vi "FinishMessage.vi"(4 "error":string="ERROR", 5 "no error":string="OK", 6 "error in":errorcluster, 9 "MessageBox in":refnum<class "MessageBox.lvclass">) -> (0 "error out":errorcluster, 3 "MessageBox out":refnum<class "MessageBox.lvclass">)   [LabVIEW 2014, in "MessageBox.lvclass"]
uses:
  MessageBox.lvclass
  MessageBox.lvclass/MessageBox.ctl
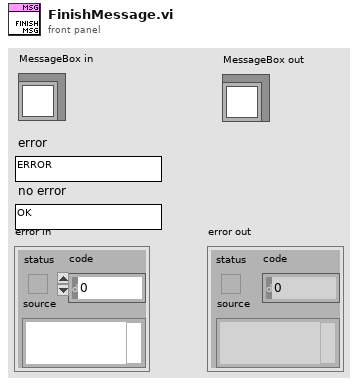
[diagram p1: front panel]
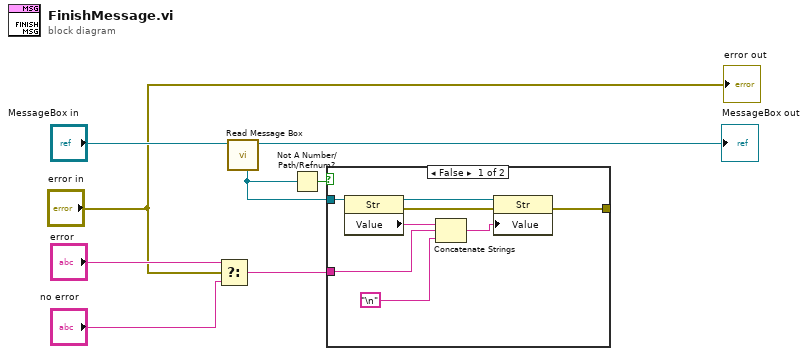
[diagram p0: block diagram]
diagram:
  n1 = Select(t="error", s="error in", f="no error") -> (s? t:f=w3:string)
  n2 = call "Read Message Box.vi"("MessageBox in"="MessageBox in") -> ("MessageBox out"=→"MessageBox out":refnum<class "MessageBox.lvclass">, "Message Box"=w5:refnum<vi>)  [unwired: 7 in]
  n3 = Not A Number/Path/Refnum?(number/path/refnum=w5) -> (NaN/Path/Refnum?=w6:bool)
  n4 = case shown="False" w6 {
    tunnel: w5 -> [w16 _]
    tunnel: w3 -> [w14 _]
    tunnel: [w10 _] -> _
    frame False {
      n5 = property class="Str"(reference=w16) -> (reference out=w12:refnum<vi>, error out=w13:errorcluster, "Value"=w15:string)  [unwired: 1 in]
      n6 = Concatenate Strings(w15, w14, "\n") -> (w11:string)
      n7 = property class="Str"(reference=w12, error in=w13, "Value"=w11) -> (error out=w10:errorcluster)  [unwired: 1 out]
    }
    frame True {
    }
  }
  "error out" <- "error in"
